vi "Conditon Tag Update.vi"(7 "L1 Prime":bool, 8 "error in (no error)":T1, 9 "OK?":bool, 10 "Panel Close?":bool, 11 "Array":T2[](array[typedef])) -> (0 "error out":T1)   [LabVIEW 2018]
uses:
  CTL/Tags.ctl
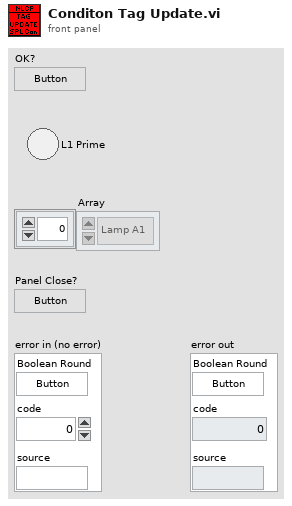
[diagram p1: front panel]
types:
  T1 = cluster{"Boolean Round":bool, "code":i32, "source":string}
  T2 = typedef "Tags.ctl" = enum16{"Lamp A1", "Lamp B1", "Lamp C1", "Lamp D1", "Lamp E1", "Lamp F1", "Lamp G1", "Lamp H1", "Lamp A2", "Lamp B2", "Lamp C2", "Lamp D2", "Lamp E2", "Lamp F2", "Lamp G2", "Lamp H2", "Ack A1", "Ack B1", "Ack C1", "Ack D1", "Ack E1", "Ack F1", "Ack G1", "Ack H1", "Ack A2", "Ack B2", "Ack C2", "Ack D2", "Ack E2", "Ack F2", "Ack G2", "Ack H2", "SSM", "SAS", "LSM", ""}
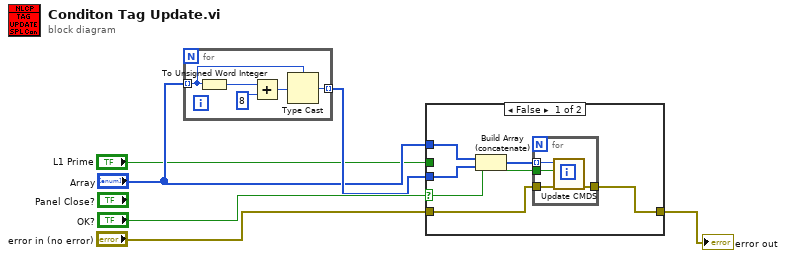
[diagram p0: block diagram]
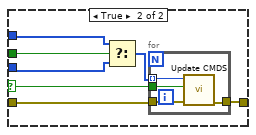
[diagram p2: hidden frame]
diagram:
  n1 = for {
    tunnel: "Array" -> [w8] mode=indexing
    tunnel: [w7] -> w5 mode=indexing
    n2 = To Unsigned Word Integer(number=w8) -> (unsigned 16bit integer=w9:u16)
    n3 = Add(x=w9, y=u16 8) -> (x+y=w11:u16)
    n4 = Type Cast(type=w8, x=w11) -> (*(type *) &x=w7:T2)
  }
  n5 = case shown="False" "OK?" {
    selector: "OK?" -> [w12 w28]
    tunnel: "error in (no error)" -> [w16 w27]
    tunnel: [w15 w26] -> w2
    tunnel: "Array" -> [w14 w25]
    tunnel: w5 -> [w13 w24]
    tunnel: "L1 Prime" -> [_ w22]
    frame False {
      n6 = Build Array (concatenate)(w14, w13) -> (w17:T2[])
      n7 = for {
        tunnel: w17 -> [w19] mode=indexing
        tunnel: w16 -> [w21]
        tunnel: [w20] -> w15
        tunnel: w12 -> [w18]
        n8 = call "Update CMDS.vi"("error in (no error)"=w21, "New Value"=w18, "Tag"=w19) -> ("error out"=w20:errorcluster)  [unwired: 8 in]
      }
    }
    frame True {
      n9 = Select(t=w25, s=w22, f=w24) -> (s? t:f=w23:T2[])
      n10 = for {
        tunnel: w28 -> [w32]
        tunnel: w27 -> [w31]
        tunnel: [w30] -> w26
        tunnel: w23 -> [w29] mode=indexing
        n11 = call "Update CMDS.vi"("error in (no error)"=w31, "New Value"=w32, "Tag"=w29) -> ("error out"=w30:errorcluster)  [unwired: 8 in]
      }
    }
  }
  "error out" <- w2
